vi "readEnobio.vi"(8 "error in (no error)":errorcluster, 9 "nSamples":i32=20, 10 "nChannels":i32=8, 11 "connection ID":refnum<k5>) -> (0 "error out":errorcluster, 2 "output array":i32[][](array[numeric]), 3 "connection ID out":refnum<k5>)   [LabVIEW 2013]
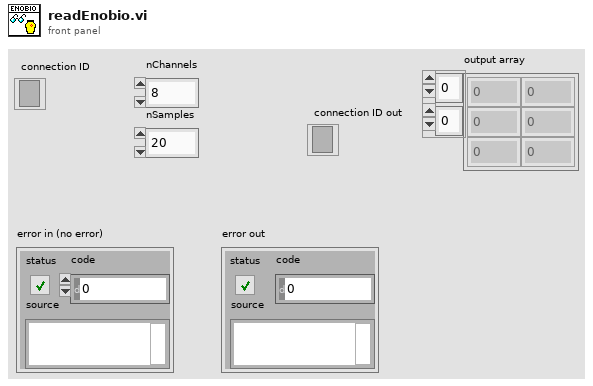
[diagram p1: front panel]
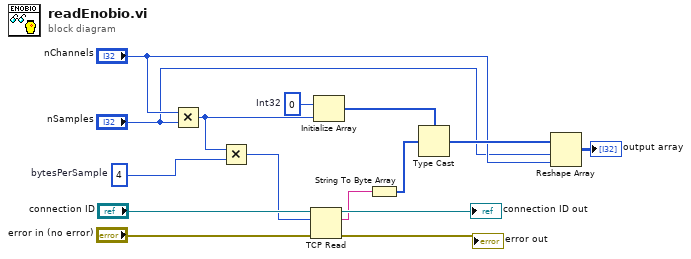
[diagram p0: block diagram]
diagram:
  w7 = 0  # Int32
  w9 = 4  # bytesPerSample
  n1 = Multiply(x="nChannels", y="nSamples") -> (x*y=w6:i32)
  n2 = Multiply(x=w6, y=w9) -> (x*y=w13:i32)
  n3 = TCP Read(connection ID="connection ID", bytes to read=w13, error in (no error)="error in (no error)") -> (connection ID out=→"connection ID out":refnum<k5>, data out=w10:string, error out=→"error out":errorcluster)  [unwired: 2 in]
  n4 = Initialize Array(w7, w6) -> (w5:i32[])
  n5 = String To Byte Array(string=w10) -> (unsigned byte array=w8:u8[])
  n6 = Type Cast(type=w5, x=w8) -> (*(type *) &x=w4:i32[])
  n7 = Reshape Array(w4, "nSamples", "nChannels") -> (→"output array":i32[][])
